vi "Cluster Exercise.vi"() -> ()   [LabVIEW 2015]
panel:
  out "Small Cluster":cluster{"Boolean":bool, "Slide Value":dbl}
  out "Modified Cluster":T1 {"Slide" scale=0.0..10.0}
  in  "Cluster":T1 {"Slide" scale=0.0..10.0}
  out "Boolean":bool
  out "Numeric":dbl
  in  "stop":bool
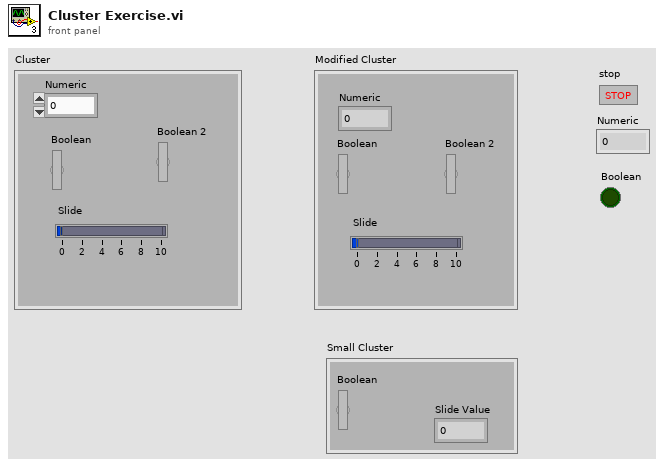
[diagram p1: front panel]
types:
  T1 = cluster{"Numeric":dbl, "Boolean":bool, "Boolean 2":bool, "Slide":dbl}
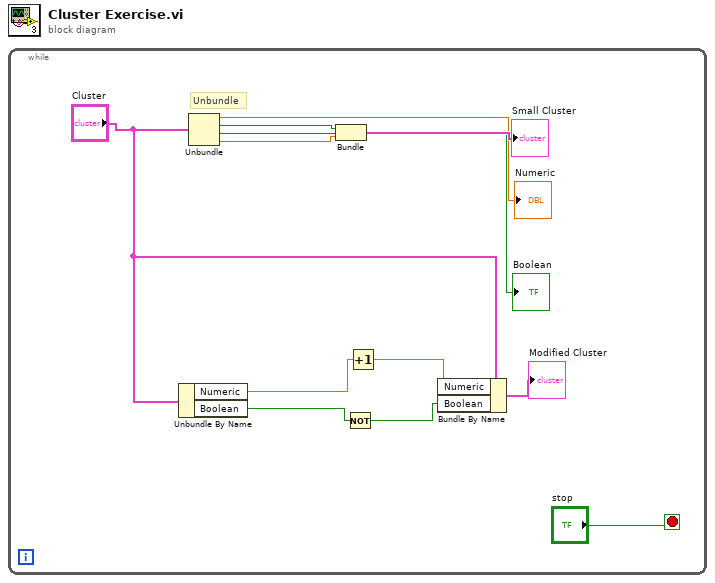
[diagram p0: block diagram]
diagram:
  n1 = while {
    stop <- "stop" stop-if-true
    # "Unbundle"
    n2 = Unbundle By Name "Unbundle By Name"("Cluster") -> ("Numeric"=w6:dbl, "Boolean"=w5:bool)
    n3 = Unbundle("Cluster") -> ("Numeric"=→"Numeric":dbl, "Boolean"=w12:bool, "Boolean 2"=→"Boolean":bool, "Slide"=w11:dbl)
    n4 = Bundle("Boolean"=w12, "Slide"=w11) -> (→"Small Cluster":cluster{"Boolean":bool, "Slide":dbl})  [unwired: 1 in]
    n5 = Not(x=w5) -> (.not. x?=w2:bool)
    n6 = Increment(x=w6) -> (x+1=w4:dbl)
    n7 = Bundle By Name "Bundle By Name"(cluster="Cluster", "Numeric"=w4, "Boolean"=w2) -> (→"Modified Cluster":T1)
  }
